vi "match.vi"() -> ()   [LabVIEW 2018]
panel:
  out "Number of iterations":dbl
  in  "Number to match":dbl
  out "Current Number":dbl
  out "Time to match":dbl
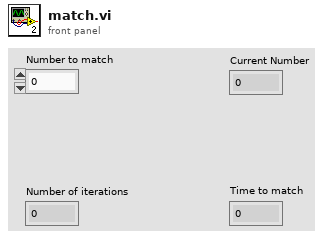
[diagram p1: front panel]
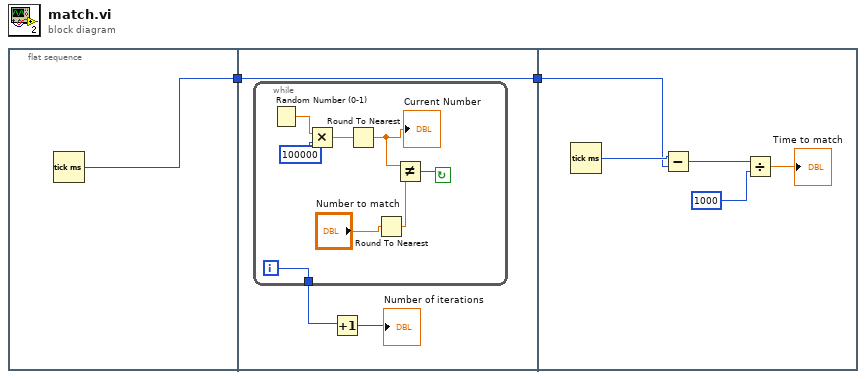
[diagram p0: block diagram]
diagram:
  n1 = flat-sequence {
    tunnel: [w3] -> w1
    tunnel: [w6] -> w2
    tunnel: w1 -> [w6]
    tunnel: w2 -> [w18]
    frame #0 {
      n2 = Tick Count (ms)() -> (millisecond timer value=w3:u32)
    }
    frame #1 {
      n3 = while {
        tunnel: [w7] -> w5
        i -> [w7]
        stop <- w12 continue-if-true
        n4 = Random Number (0-1)() -> (number: 0 to 1=w13:dbl)
        n5 = Multiply(x=w13, y=100000) -> (x*y=w14:dbl)
        n6 = Round To Nearest(number=w14) -> (nearest integer value=w11:dbl)
        "Current Number" <- w11
        n7 = Round To Nearest(number="Number to match") -> (nearest integer value=w10:dbl)
        n8 = Not Equal?(x=w11, y=w10) -> (x != y?=w12:bool)
      }
      n9 = Increment(x=w5) -> (x+1=→"Number of iterations":i32)
    }
    frame #2 {
      n10 = Tick Count (ms)() -> (millisecond timer value=w19:u32)
      n11 = Subtract(x=w19, y=w18) -> (x-y=w17:u32)
      n12 = Divide(x=w17, y=1000) -> (x/y=→"Time to match":dbl)
    }
  }
